vi "initialise.vi"(8 "error in (no error)":errorcluster, 11 "ScanModeMG091111IntrinsicImaging in":refnum<class "ImagingModeMG091111IntrinsicImaging.lvclass">) -> (0 "error out":errorcluster, 3 "ScanModeMG091111IntrinsicImaging out":refnum<class "ImagingModeMG091111IntrinsicImaging.lvclass">)   [LabVIEW 2010, in "ImagingModeMG091111IntrinsicImaging.lvclass"]
doc: "The dynamic dispatch-version of this VI initalises the plug-in object by allocating and initalising any dynamic resources need."
uses:
  ImagingModeMG091111IntrinsicImaging.lvclass
  ImagingModeDL091001Scaffold/ImagingModeDL091001Scaffold/ImagingModeDL091001Scaffold.lvclass
  ScanHead/GenericScanHead/GenericScanHead/GenericScanHead.lvclass
  Instrument/GenericInstrument/GenericInstrument/GenericInstrument.lvclass
  Stimulator/GenericStimulator/GenericStimulator/GenericStimulator.lvclass
  Display/GenericDisplay/GenericDisplay/GenericDisplay.lvclass
  Analyser/GenericAnalyser/GenericAnalyser/GenericAnalyser.lvclass
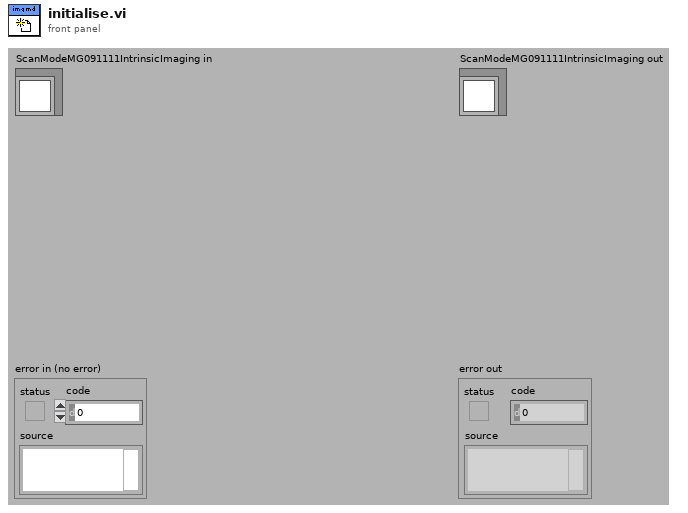
[diagram p1: front panel]
types:
  T1 = enum8{"Enabled", "Disabled", "Disabled and Grayed Out"}
  T2 = typedef "controls_refs.ctl" = cluster{"scan start button":refnum<vi>, "tabs":cluster{"main":refnum<vi>, "settings":refnum<vi>}, "subpanels":cluster{"imagingMode":refnum<vi>, "scanHead":refnum<vi>, "display":refnum<vi>, "experimentController":refnum<vi>, "instrument":refnum<vi>, "stage":refnum<vi>, "stimulator":refnum<vi>, "dataCollection":refnum<vi>, "analyser":refnum<vi>, "daq":refnum<vi>, "imageAssembler":refnum<vi>}, "drop-downs":cluster{"run mode":refnum<vi>, "imagingMode":refnum<vi>, "experimentalController":refnum<vi>, "objective":refnum<vi>}, "status lights":cluster{"experimentController":refnum<vi>, "imagingMode":refnum<vi>, "scanHead":refnum<vi>, "daq":refnum<vi>, "imageAssembler":refnum<vi>, "dataCollection":refnum<vi>, "display":refnum<vi>, "analyser":refnum<vi>, "stage":refnum<vi>, "stimulator":refnum<vi>, "instrument":refnum<vi>}, "message":refnum<vi>, "stimulator enabled?":refnum<vi>, "saving":cluster{"data folder path":refnum<vi>, "file base name":refnum<vi>, "notebook":refnum<vi>}, "progress bar":refnum<vi>, "update icon":refnum<vi>, "title":refnum<vi>, "main vi":refnum<vi>, "user":refnum<vi>, "exit_button":refnum<vi>, "CPU usage %":refnum<vi>}
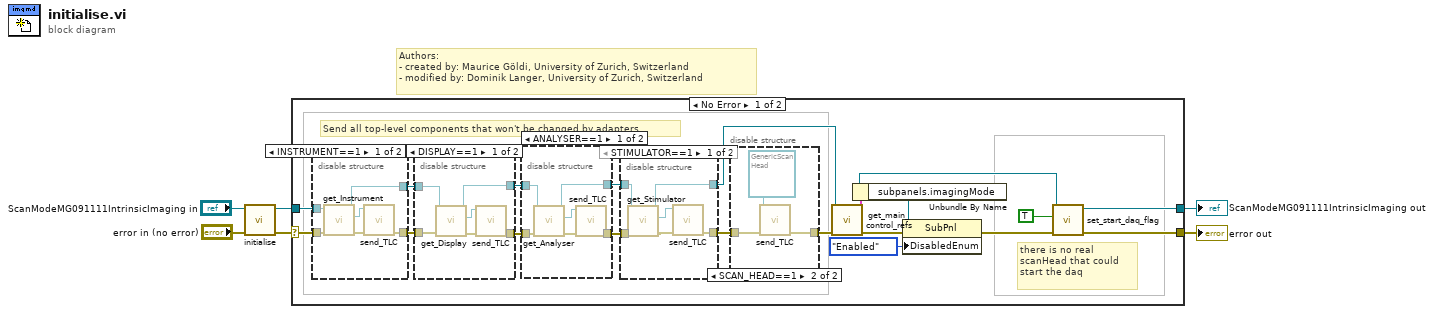
[diagram p0: block diagram]
diagram:
  # "Authors: \n- created by: Maurice Göldi, University of Zurich, Switzerland\n- modified by: Dominik Langer, University of Zurich, Switzerland"
  n1 = call-parent "initialise.vi"("error in (no error)"="error in (no error)", "GenericPlugin in"="ScanModeMG091111IntrinsicImaging in") -> ("error out"=w1:errorcluster, "GenericPlugin out"=w3:refnum<class "ImagingModeMG091111IntrinsicImaging.lvclass">)  [unwired: 8 in]
  n2 = case shown="No Error" w1 {
    selector: w1 -> [w25 w63]
    tunnel: [w8 w63] -> w4
    tunnel: w3 -> [w26 w64]
    tunnel: [w7 w64] -> w2
    frame No Error {
      # "there is no real scanHead that could start the daq"
      # "Send all top-level components that won't be changed by adapters..."
      n3 = disable-structure shown="INSTRUMENT==1" {
        disable-tunnel: w26 -> [w60 w61]
        disable-tunnel: w25 -> [w59 w62]
        disable-tunnel: [w58 w61] -> w12
        disable-tunnel: [w56 w62] -> w13
        frame condition #0 {
          n4 = call-dynamic "get_Instrument.vi"("error in (no error)"=w59, "ScanModeDL090923Scaffold in"=w60) -> ("error out"=w57:errorcluster, "Instrument"=w55:refnum<class "GenericInstrument.lvclass">, "ScanModeDL090923Scaffold out"=w58:refnum<class "ImagingModeMG091111IntrinsicImaging.lvclass">)  [unwired: 4 in, 3 out]
          n5 = call-dynamic "send_TLC.vi"("error in (no error)"=w57, "GenericToplevelComponent in"=w55) -> ("error out"=w56:errorcluster)  [unwired: 8 in, 1 out]
        }
        frame condition #1 (active) {
        }
      }
      n6 = disable-structure shown="DISPLAY==1" {
        disable-tunnel: w12 -> [w52 w53]
        disable-tunnel: [w51 w53] -> w24
        disable-tunnel: w13 -> [w50 w54]
        disable-tunnel: [w48 w54] -> w22
        frame condition #0 {
          n7 = call-dynamic "get_Display.vi"("error in (no error)"=w50, "ScanModeDL090923Scaffold in"=w52) -> ("error out"=w49:errorcluster, "Display"=w47:refnum<class "GenericDisplay.lvclass">, "ScanModeDL090923Scaffold out"=w51:refnum<class "ImagingModeMG091111IntrinsicImaging.lvclass">)  [unwired: 4 in, 3 out]
          n8 = call-dynamic "send_TLC.vi"("error in (no error)"=w49, "GenericToplevelComponent in"=w47) -> ("error out"=w48:errorcluster)  [unwired: 8 in, 1 out]
        }
        frame condition #1 (active) {
        }
      }
      n9 = disable-structure shown="ANALYSER==1" {
        disable-tunnel: w24 -> [w44 w45]
        disable-tunnel: [w43 w45] -> w23
        disable-tunnel: w22 -> [w42 w46]
        disable-tunnel: [w40 w46] -> w21
        frame condition #0 {
          n10 = call-dynamic "get_Analyser.vi"("error in (no error)"=w42, "ScanModeDL090923Scaffold in"=w44) -> ("error out"=w41:errorcluster, "Analyser"=w39:refnum<class "GenericAnalyser.lvclass">, "ScanModeDL090923Scaffold out"=w43:refnum<class "ImagingModeMG091111IntrinsicImaging.lvclass">)  [unwired: 4 in, 3 out]
          n11 = call-dynamic "send_TLC.vi"("error in (no error)"=w41, "GenericToplevelComponent in"=w39) -> ("error out"=w40:errorcluster)  [unwired: 8 in, 1 out]
        }
        frame condition #1 (active) {
        }
      }
      n12 = disable-structure shown="STIMULATOR==1" {
        disable-tunnel: w23 -> [w36 w38]
        disable-tunnel: w21 -> [w35 w37]
        disable-tunnel: [w33 w37] -> w20
        disable-tunnel: [w31 w38] -> w18
        frame condition #0 {
          n13 = call-dynamic "get_Stimulator.vi"("error in (no error)"=w35, "ScanModeDL090923Scaffold in"=w36) -> ("error out"=w34:errorcluster, "Stimulator"=w32:refnum<class "GenericStimulator.lvclass">, "ScanModeDL090923Scaffold out"=w31:refnum<class "ImagingModeMG091111IntrinsicImaging.lvclass">)  [unwired: 4 in, 3 out]
          n14 = call-dynamic "send_TLC.vi"("error in (no error)"=w34, "GenericToplevelComponent in"=w32) -> ("error out"=w33:errorcluster)  [unwired: 8 in, 1 out]
        }
        frame condition #1 (active) {
        }
      }
      n15 = disable-structure shown="SCAN_HEAD==1" {
        disable-tunnel: w20 -> [w27 w29]
        disable-tunnel: [w27 w28] -> w19
        frame condition #0 (active) {
        }
        frame condition #1 {
          n16 = call-dynamic "send_TLC.vi"("error in (no error)"=w29, "GenericToplevelComponent in"=refnum<class "GenericScanHead.lvclass"> refnum ("GenericScanHead.lvclass")) -> ("error out"=w28:errorcluster)  [unwired: 8 in, 1 out]
        }
      }
      n17 = call-dynamic "get_main_control_refs.vi"("error in (no error)"=w19, "GenericPlugin.lvclass in"=w18) -> ("error out"=w16:errorcluster, "control references"=w17:T2, "GenericPlugin.lvclass out"=w10:refnum<class "ImagingModeMG091111IntrinsicImaging.lvclass">)  [unwired: 7 in]
      n18 = Unbundle By Name(w17) -> ("subpanels.imagingMode"=w15:refnum<vi>)
      n19 = property class="SubPnl"(reference=w15, error in=w16, "DisabledEnum"=T1."Enabled" ("Disabled")) -> (error out=w11:errorcluster)  [unwired: 1 out]
      n20 = call-dynamic "set_start_daq_flag.vi"("error in (no error)"=w11, "start daq from within imagingMode?"=TRUE, "ImagingModeDL090923Scaffold in"=w10) -> ("error out"=w8:errorcluster, "ImagingModeDL090923Scaffold out"=w7:refnum<class "ImagingModeMG091111IntrinsicImaging.lvclass">)  [unwired: 7 in]
    }
    frame Error {
    }
  }
  "error out" <- w4
  "ScanModeMG091111IntrinsicImaging out" <- w2
